vi "Get Registered Notifiers.vi"(8 "error in (no error)":errorcluster) -> (0 "error out":errorcluster, 3 "Notifier References":refnum<notifier>[](array[refnum]))   [LabVIEW 2021]
doc: "This VI returns an array of references for every queue that is registered in the Queue Registry."
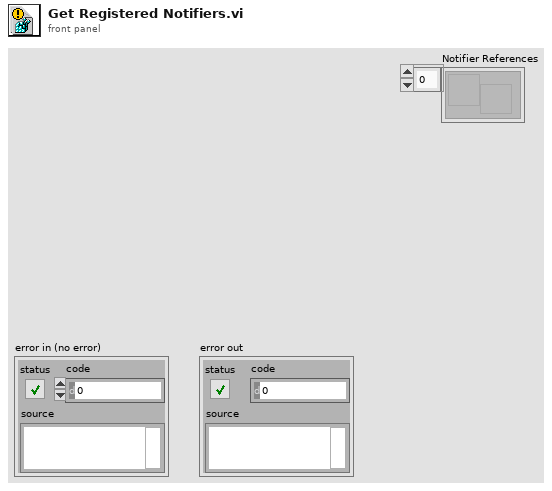
[diagram p1: front panel]
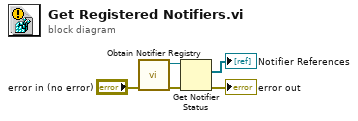
[diagram p0: block diagram]
diagram:
  n1 = call "Obtain Notifier Registry.vi"("error in (no error)"="error in (no error)") -> ("error out"=w3:errorcluster, "Notifier Registry"=w2:refnum<notifier>)  [unwired: 9 in]
  n2 = Get Notifier Status(notifier=w2, error in (no error)=w3) -> (current notification=→"Notifier References":refnum<notifier>[], error out=→"error out":errorcluster)  [unwired: 3 out]
